vi "Get state.vi"(8 "error in (no error)":errorcluster, 11 "StateManager in":refnum<class "StateManager.lvclass">) -> (0 "error out":errorcluster, 1 "previousState":u32, 2 "currentState":u32, 3 "StateManager out":refnum<class "StateManager.lvclass">, 4 "overflow":bool, 5 "timeout":bool)   [LabVIEW 2018, in "StateManager.lvclass"]
uses:
  StateManager.lvclass
  StateManager.lvclass/StateManager.ctl
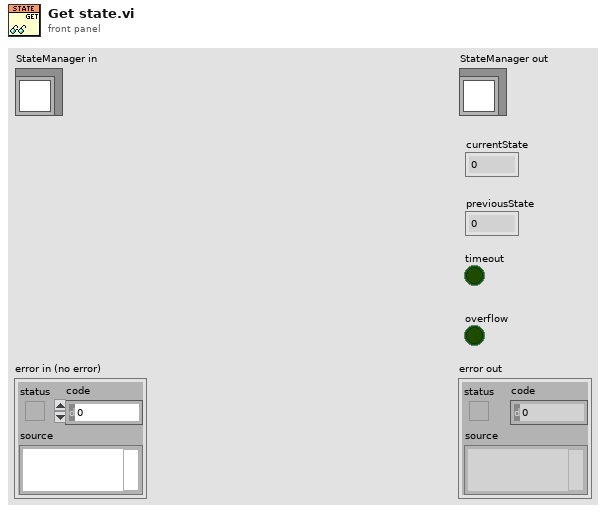
[diagram p1: front panel]
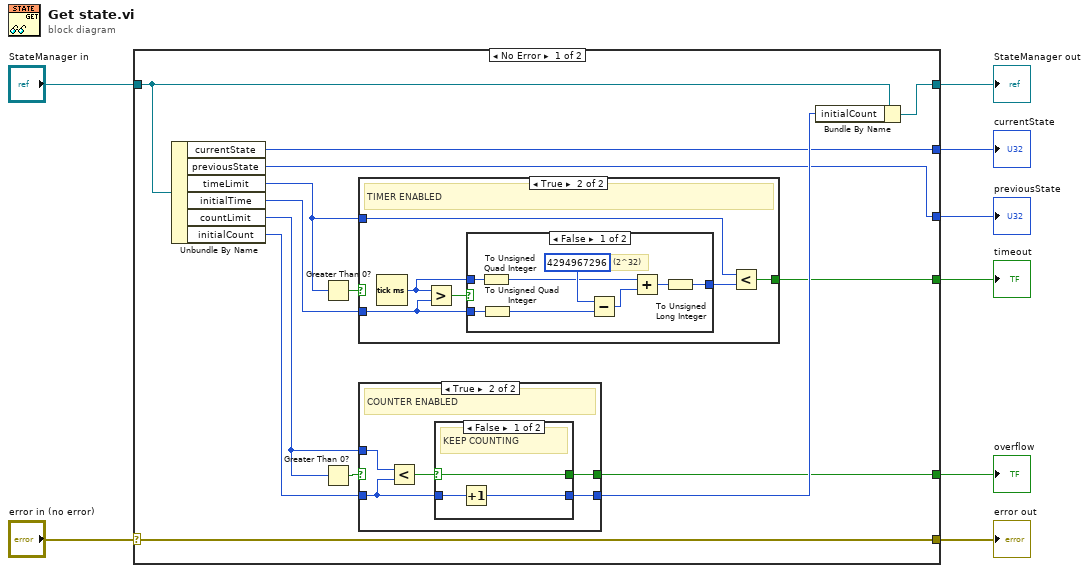
[diagram p0: block diagram]
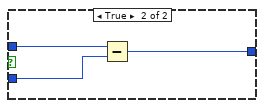
[diagram p3: hidden frame]
diagram:
  n1 = case shown="No Error" "error in (no error)" {
    selector: "error in (no error)" -> [w9 w53]
    tunnel: [w9 w53] -> w7
    tunnel: [w14 w54] -> w5
    tunnel: "StateManager in" -> [w16 w54]
    tunnel: [w11 _] -> w4
    tunnel: [w10 _] -> w3
    tunnel: [w13 _] -> w2
    tunnel: [w12 _] -> w1
    frame No Error {
      n2 = Unbundle By Name(w16) -> ("currentState"=w11:u32, "previousState"=w10:u32, "timeLimit"=w17:u32, "initialTime"=w18:u32, "countLimit"=w20:u32, "initialCount"=w21:u32)
      n3 = Greater Than 0?(x=w17) -> (x > 0?=w19:bool)
      n4 = Greater Than 0?(x=w20) -> (x > 0?=w22:bool)
      n5 = case shown="True" w19 {
        selector: w19 -> [w23 _]
        tunnel: w18 -> [_ w28]
        tunnel: w17 -> [_ w26]
        tunnel: [w23 w24] -> w12
        frame False {
          # "TIMER DISABLED"
        }
        frame True {
          # "TIMER ENABLED"
          n6 = Tick Count (ms)() -> (millisecond timer value=w27:u32)
          n7 = Greater?(x=w27, y=w28) -> (0:w29:bool)
          n8 = case shown="False" w29 {
            tunnel: w28 -> [w37 w38]
            tunnel: w27 -> [w36 w39]
            tunnel: [w30 w40] -> w25
            frame False {
              # "(2^32)"
              n9 = To Unsigned Quad Integer(1:w36) -> (0:w32:u64)
              n10 = To Unsigned Quad Integer(1:w37) -> (0:w35:u64)
              n11 = Subtract(x=u64 4294967296 ("initial Tick"), y=w35) -> (x-y=w33:u64)
              n12 = Add(x=w32, y=w33) -> (x+y=w31:u64)
              n13 = To Unsigned Long Integer(number=w31) -> (unsigned 32bit integer=w30:u32)
            }
            frame True {
              n14 = Subtract(x=w39, y=w38) -> (x-y=w40:u32)
            }
          }
          n15 = Less?(x=w26, y=w25) -> (x < y?=w24:bool)
        }
      }
      n16 = case shown="True" w22 {
        selector: w22 -> [w42 _]
        tunnel: w21 -> [w41 w45]
        tunnel: w20 -> [_ w47]
        tunnel: [w42 w44] -> w13
        tunnel: [w41 w43] -> w15
        frame False {
          # "COUNTER DISABLED"
        }
        frame True {
          # "COUNTER ENABLED"
          n17 = Less?(x=w47, y=w45) -> (x < y?=w46:bool)
          n18 = case shown="False" w46 {
            selector: w46 -> [w50 w52]
            tunnel: [w50 w52] -> w44
            tunnel: w45 -> [w49 w51]
            tunnel: [w48 w51] -> w43
            frame False {
              # "KEEP COUNTING"
              n19 = Increment(x=w49) -> (x+1=w48:u32)
            }
            frame True {
              # "COUNTER OVERFLOW"
            }
          }
        }
      }
      n20 = Bundle By Name(cluster=w16, "initialCount"=w15) -> (w14:refnum<class "StateManager.lvclass">)
    }
    frame Error {
    }
  }
  "error out" <- w7
  "StateManager out" <- w5
  "currentState" <- w4
  "previousState" <- w3
  "overflow" <- w2
  "timeout" <- w1
